vi "Variable Z Script (old).vi"() -> ()   [LabVIEW 2010]
uses:
  <vilib>/Utility/file.llb/Write To Spreadsheet File (string).vi
panel:
  in  "Strain Points":T1
  in  "Values":string[](array[string])=["Structure ID", "Structure Name"]
  in  "Headers":string[](array[string])=["Structure ID", "Structure Name"]
  in  "Periodicity":string="A3B12"
  in  "Folder Prefix Name":string="A3B12_Lamallar"
  in  "Strain Directory":path=path "D:/Ab-initio/VASP Calcs/2D_Grain Boundaries/Batch25_20130914"
  in  "Structure Name":string="A3B12_Lamallar"
  in  "Structure File":path=path "D:/Ab-initio/VASP Calcs/2D_Grain Boundaries/Batch18_20130828/A3B12_Periodic_Twin/CONTCAR"
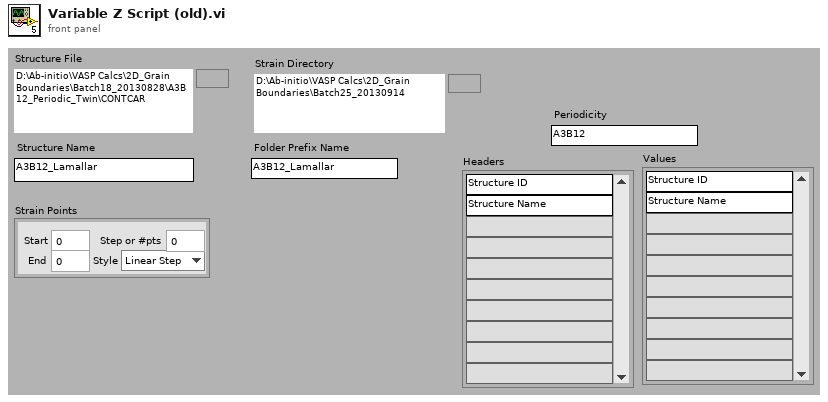
[diagram p1: front panel]
types:
  T1 = cluster{"Start":dbl, "End":dbl, "Step or #pts":dbl, "Style":enum16{"Linear Step", "Linear Pts", "Log Pts"}}
  T2 = cluster{"Structure Name":string, "Lattice vector a":dbl[], "Lattice vector b":dbl[], "Lattice vector c":dbl[], "Atoms Array":cluster{"Atom Name":string, "Positions (Direct)":dbl[][], "Positions (Cartesian)":dbl[][]}[], "# of atoms":i32}
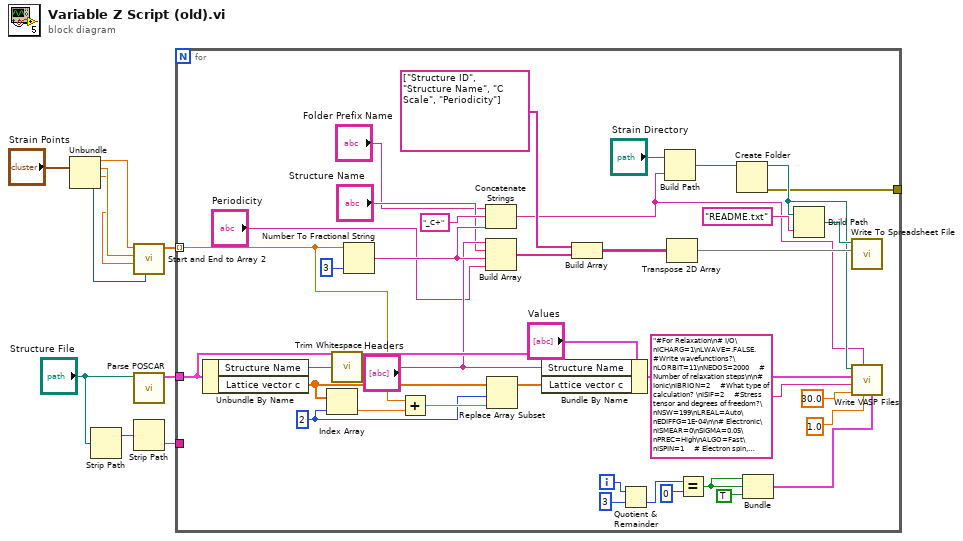
[diagram p0: block diagram]
diagram:
  n1 = Unbundle("Strain Points") -> ("Start"=w4:dbl, "End"=w3:dbl, "Step or #pts"=w2:dbl, "Style"=w1:enum16{"Linear Step", "Linear Pts", "Log Pts"})
  n2 = Strip Path(path="Structure File") -> (stripped path=w8:path)  [unwired: 1 out]
  n3 = call "Start and End to Array 2.vi"("Sweep Style"=w1, "Step or # Pts"=w2, "End"=w3, "Start"=w4) -> ("Array"=w10:dbl[])  [unwired: 7 in]
  n4 = call "Parse POSCAR.vi"("POSCAR File"="Structure File") -> ("Structure"=w6:T2)  [unwired: 7 in, 3 out]
  n5 = Strip Path(path=w8) -> (name=w7:string)  [unwired: 1 out]
  n6 = for {
    tunnel: w6 -> [w46]
    tunnel: w10 -> [w44] mode=indexing
    tunnel: w7 -> [_]
    tunnel: [w32] -> _
    i -> [w26]
    w15 = 2 ("index")
    n7 = Unbundle By Name(w46) -> ("Structure Name"=w30:string, "Lattice vector c"=w16:dbl[])
    n8 = Index Array(array=w16, index=w15) -> (element=w18:dbl)
    n9 = call <vilib>:"Trim Whitespace.vi"("string"=w30) -> ("trimmed string"=w28:string)  [unwired: 1 in]
    n10 = Number To Fractional String(number=w44, precision (6)=i16 3) -> (F-format string=w29:string)  [unwired: 2 in]
    n11 = Add(x=w44, y=w18) -> (x+y=w17:dbl)
    n12 = Concatenate Strings("Folder Prefix Name", "_C+" ("string"), w29) -> (w27:string)
    n13 = Build Array(w28, "Structure Name", w29, "Periodicity") -> (w31:string[])
    n14 = Replace Array Subset(array=w16, new element=w17, index=w15) -> (w14:dbl[])
    n15 = Bundle By Name(cluster=w46, "Structure Name"=w28, "Lattice vector c"=w14) -> (w45:T2)
    n16 = Build Array(string[] ["Structure ID", "Structure Name", "C Scale", "Periodicity"] ("element"), w31) -> (w40:string[][])
    n17 = Quotient & Remainder(x=w26, y=3) -> (floor(x/y)=w25:i32)  [unwired: 1 out]
    n18 = Build Path(base path="Strain Directory", name or relative path=w27) -> (appended path=w34:path)
    n19 = Transpose 2D Array(2D array=w40) -> (transposed array=w39:string[][])
    n20 = Equal?(x=w25, y=0) -> (x = y?=w22:bool)
    n21 = Create Folder(path (use dialog)=w34) -> (created path=w33:path, error out=w32:errorcluster)  [unwired: 2 in, 1 out]
    n22 = Bundle(w22, w22, TRUE) -> (w20:cluster{bool, bool, bool})  [unwired: 1 in]
    n23 = Build Path(base path=w33, name or relative path="README.txt") -> (appended path=w42:path)
    n24 = call-poly <vilib>:"Write To Spreadsheet File.vi"("2D data"=w39, "file path (dialog if empty)"=w42) -> ()  [unwired: 6 in, 1 out]
    n25 = call "Write VASP Files.vi"("Email?"=w20, "Volume Factor"=1.0, "Submitname on Carbon"=w27, "K-Points File"=30.0 ("|G| Factor"), "INCAR File"="#For Relaxation\n# I/O\nICHARG=1\nLWAVE=.FALSE.  #Write wavefunctions?\nLORBIT=11\nNEDOS=2000     # Number of relaxation steps\n\n# Ionic\nIBRION=2     #What type of calculation? \nISIF=2     #Stress tensor and degrees of freedom?\nNSW=199\nLREAL=Auto\nEDIFFG=1E-04\n\n# Electronic\nISMEAR=0\nSIGMA=0.05\nPREC=High\nALGO=Fast\nISPIN=1     # Electron spin, 1=nope, 2=account for spin\nNELM=100\nNELMIN=5\nEDIFF=1E-06    #energy difference to stop relaxation at\n\n# Parallelization\nNPAR=4     # change this to the number of nodes in the job\n", "Atomic Structure"=w45, "Path to place files into"=w33) -> ()  [unwired: 5 in]
  }
